vi "CRYPEAQ SpreadCB.vi"(10 "Center Frequency":dbl[](array[numeric]), 11 "E":dbl[](array[numeric])) -> (2 "B":dbl[](array[numeric]), 3 "Es":dbl[](array[numeric]))   [LabVIEW 2013]
panel:
  out "XY Graph 4":cluster{"Center Frequency":dbl[], "Es":dbl[]}[](graph)
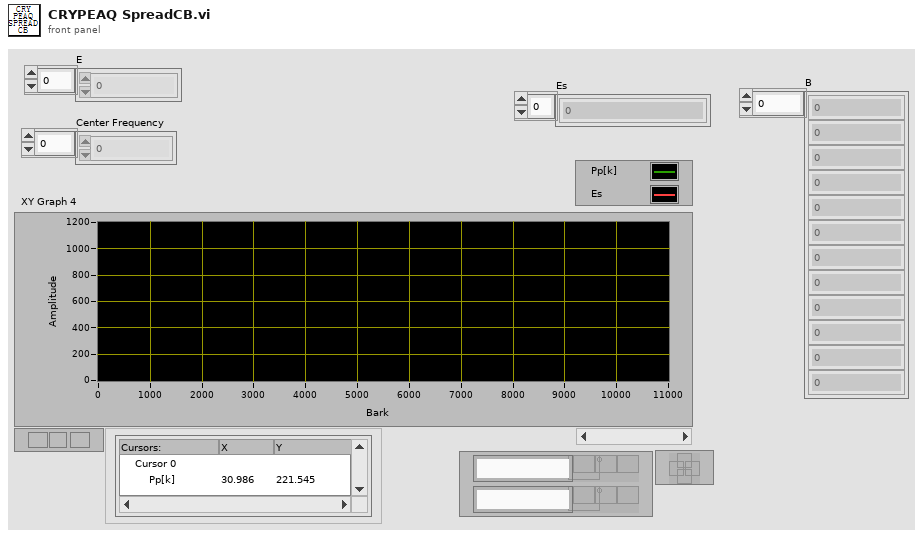
[diagram p1: front panel]
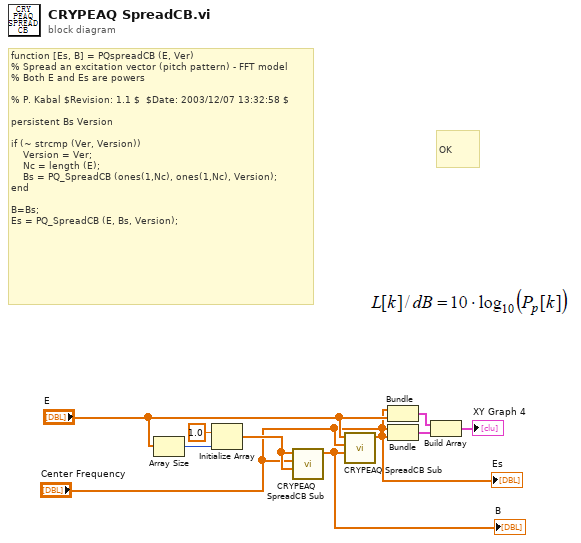
[diagram p0: block diagram]
diagram:
  # "OK"
  # "function [Es, B] = PQspreadCB (E, Ver)\n% Spread an excitation vector (pitch pattern) - FFT model\n% Both E and Es are powers\n\n% P. Kabal $Revision: 1.1 $  $Date: 2003/12/07 13:32:58 $\n\npersistent Bs Version\n\nif (~ strcmp (Ver, Version))\n    Version = Ver;\n    Nc = length (E);\n    Bs = PQ_SpreadCB (ones(1,Nc), ones(1,Nc), Version);\nend\n\nB=Bs;\nEs = PQ_SpreadCB (E, Bs, Version);"
  n1 = Array Size(array="E") -> (size(s)=w1:i32)
  n2 = Initialize Array(1.0 ("element"), w1) -> (w9:dbl[])
  n3 = call "CRYPEAQ SpreadCB Sub.vi"("Bs"=w9, "Center Frequency"="Center Frequency", "E"=w9) -> ("Es"=w2:dbl[])  [unwired: 8 in]
  "B" <- w2
  n4 = call "CRYPEAQ SpreadCB Sub.vi"("Bs"=w2, "Center Frequency"="Center Frequency", "E"="E") -> ("Es"=w7:dbl[])  [unwired: 8 in]
  "Es" <- w7
  n5 = Bundle("Center Frequency"="Center Frequency", "E"="E") -> (w4:cluster{"Center Frequency":dbl[], "E":dbl[]})  [unwired: 1 in]
  n6 = Bundle("Center Frequency"="Center Frequency", "Es"=w7) -> (w5:cluster{"Center Frequency":dbl[], "Es":dbl[]})  [unwired: 1 in]
  n7 = Build Array(w4, w5) -> (→"XY Graph 4":cluster{"Center Frequency":dbl[], "Es":dbl[]}[])
